vi "Ball Pick Up.vi"(6 "Ball Y":dbl, 7 "Max Speed":dbl, 8 "Ball X":dbl, 9 "Yaw":dbl=1.57, 10 "Speed Setpoint":dbl=0.4, 11 "Ball Detected":bool) -> (1 "Speed Right":dbl, 2 "Speed Left":dbl)   [LabVIEW 2015]
uses:
  Team900-VIs/Team900SwerveDrive/Team900SwerveDrive.lvlib
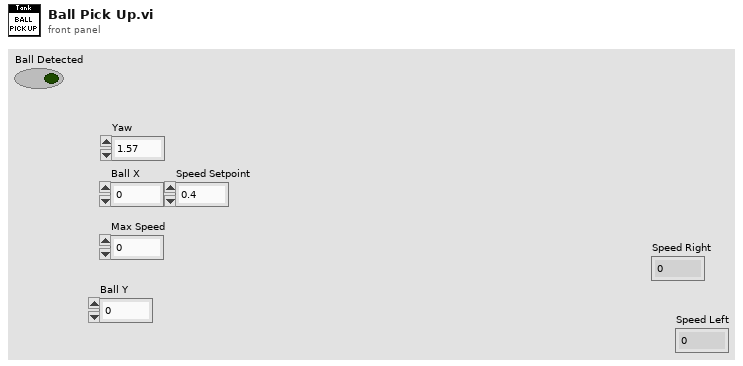
[diagram p1: front panel]
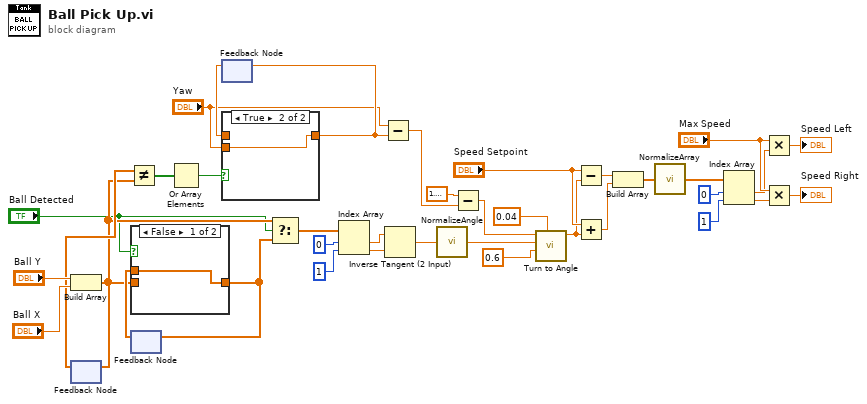
[diagram p0: block diagram]
diagram:
  n1 = Build Array("Ball Y", "Ball X") -> (w2:dbl[])
  n2 = feedback-in #1(w2) -> ()
  n3 = feedback #1() -> (w15:dbl[])  [unwired: 1 in]
  n4 = Not Equal?(x=w15, y=w2) -> (x != y?=w14:bool[])
  n5 = feedback #2() -> (w9:dbl[])  [unwired: 1 in]
  n6 = case shown="False" "Ball Detected" {
    tunnel: [w38 w39] -> w3
    tunnel: w2 -> [_ w39]
    tunnel: w9 -> [w38 _]
    frame False {
    }
    frame True {
    }
  }
  n7 = feedback-in #2(w3) -> ()
  n8 = Or Array Elements(Boolean array=w14) -> (logical OR=w13:bool)
  n9 = feedback #3() -> (w34:dbl)  [unwired: 1 in]
  n10 = case shown="True" w13 {
    tunnel: [w40 w41] -> w33
    tunnel: "Yaw" -> [_ w41]
    tunnel: w34 -> [w40 _]
    frame False {
    }
    frame True {
    }
  }
  n11 = feedback-in #3(w33) -> ()
  n12 = Select(t=w2, s="Ball Detected", f=w3) -> (s? t:f=w4:dbl[])
  n13 = Index Array(array=w4, index #1=0 ("index"), index #2=1 ("index")) -> (element #1=w6:dbl, element #2=w5:dbl)
  n14 = Subtract(x="Yaw", y=w33) -> (x-y=w12:dbl)
  n15 = Inverse Tangent (2 Input)(1:w5, 2:w6) -> (0:w37:dbl)
  n16 = call "NormalizeAngle.vi"("angle (rad)"=w37) -> ("angle (between pi and -pi)"=w28:dbl)
  n17 = Subtract(x=1.5707963267948966, y=w12) -> (x-y=w11:dbl)
  n18 = call "Turn to Angle.vi"("Angle Tolerance"=0.04, "Rotation Multiplier"=0.6, "Target angle"=w28, "Angle (radians; 0 = right)"=w11) -> ("Turn Set Point"=w29:dbl)  [unwired: 3 in, 1 out]
  n19 = Subtract(x="Speed Setpoint", y=w29) -> (x-y=w27:dbl)
  n20 = Add(x="Speed Setpoint", y=w29) -> (x+y=w20:dbl)
  n21 = Build Array(w27, w20) -> (w26:dbl[])
  n22 = call "NormalizeArray.vi"("array"=w26) -> ("normalized array"=w25:dbl[])
  n23 = Index Array(array=w25, index #1=0 ("index"), index #2=1 ("index")) -> (element #1=w22:dbl, element #2=w21:dbl)
  n24 = Multiply(x="Max Speed", y=w22) -> (x*y=→"Speed Left":dbl)
  n25 = Multiply(x="Max Speed", y=w21) -> (x*y=→"Speed Right":dbl)
